vi "11-QNET_MECHKIT_Switches_and_LEDs.vi"() -> ()   [LabVIEW 2017]
doc: "This VI is to be used with the NI-ELVIS and the QNET-Mechatronic Sensors I module. The objective is to calibrate the analog sensors."
uses:
  <vilib>/Simulation/Scripting/Companion Diagram/SimConfigNode/SimParams.ctl
  <vilib>/Simulation/Scripting/Companion Diagram/SimConfigNode/_simSolvers.ctl
  <vilib>/Simulation/Implementation/Shared/SIMSCR Execution Mode.ctl
  <vilib>/Simulation/Param Hierarchy/Typedefs/SIMPH Param Control Actions.ctl
  <vilib>/Simulation/Implementation/Shared/NILVSim_ParamChanged.vi
  <vilib>/Simulation/Implementation/Shared/NILVSIM_BeginStep.vi
  <vilib>/Simulation/SignalDisplay/Implementation/NILVSim Time Waveform.llb/SIM Time Waveform (scalar).vi
  <vilib>/Simulation/Utility/Implementation/SIM Halt.vi
  <vilib>/Simulation/Implementation/Shared/NILVSim_Manager.vi
  <vilib>/Utility/error.llb/Clear Errors.vi
  <vilib>/Simulation/Implementation/Shared/NILVSim_FinalizeModel.vi
  <vilib>/Simulation/Implementation/Shared/SIM Unbundle Sim Info.vi
  <vilib>/Simulation/Implementation/Shared/NILVSim_Initialize.vi
  QNET Library/QNET_Drivers.llb/QNET_MECHKIT_AI_Read.vi
  QNET Library/Quanser_DAQ_MX_Drivers.llb/DO_Write_Multi_MX.vi
  <vilib>/Simulation/Utility/Implementation/NILVSim Get Time and IsAcceptedStep.vi
  <vilib>/Simulation/Implementation/Shared/SIMSH Read Queue.vi
  <vilib>/Simulation/Implementation/Shared/NILVSim_GetModelError.vi
  <vilib>/Simulation/Implementation/Shared/SIM Bundle Sim Info.vi
  <vilib>/Simulation/Scripting/Companion Diagram/SimConfigNode/SimDog.xnode
  <vilib>/Simulation/Implementation/XNodeFramework/SimXNode/SimX.xnode
  <vilib>/Simulation/Implementation/Shared/NI_SIM_Implementation.lvlib
panel:
  in  "Sampling Rate (Hz)":dbl=100.0 min=0.0 max=1000.0 step=25.0 format="%.1f"
  in  "Device":tag="Dev1"
  in  "Tab Control":T1(tab)
  out "Optical Switch":waveform(dbl)(graph)
  out "Optical Switch - Digital":waveform(dbl)(graph)
  in  "Threshold":dbl(slide) min=0.0 max=5.0 step=0.05 scale=0.0..5.0
  out "Micro Switch":waveform(dbl)(graph)
  out "Micro Switch - Digital":waveform(dbl)(graph)
  in  "Gain":dbl step=0.05
  in  "Offset":dbl
  out "Push Button":waveform(dbl)(graph)
  in  "PB Offset":dbl caption="Offset"
  in  "PB Gain":dbl caption="Gain" step=0.05
  out "Push Button - Digital":waveform(dbl)(graph)
  in  "Digital Outputs":cluster{"DO 0":bool, "DO 1":bool}={"DO 0"=TRUE, "DO 1"=FALSE}
  in  "Stop":bool
  # "QNET-Switches and LEDs"
  # "NOTE: Place J7 to \"Opto Switch\", J8 to \"Micro Switch\", and J9 to \"Push Button\"."
  # "s"
  # "1) Take piece of paper and slide it up and down into the optical switch.\n2) Examine the raw responses in the \"Optical Switch\" chart.\n3) Adjust threshold to obtain on/off measurement in the \n\"Optical Switch - Digital\" chart."
  # "if (x > threshold) then y = 1\nelse y = 0"
  # "y = Gain*x + Offset\nwhere:\nx is the switch signal\ny is the processed switch signal"
  # "1) Press on Mirco Switch and examine response in \"Micro Switch\" scope.\n2) Adjust the Gain and Offset such that this signal goes from 0 to 1 \nin the \"Micro Switch - Digital\" scope when the Micro Switch is pressed."
  # "y = Gain*x + Offset\nwhere:\nx is the push button signal\ny is the processed signal"
  # "1) Press on Push Button and examine response in \"Push Button\" scope.\n2) Adjust the Gain and Offset such that the signal goes from 0 to 1 in the \n\"Push Button - Digital\" scope when the Push Button is pressed."
  # "Turn switches UP and DOWN and examine response of LEDs QNET-MECHKIT board."
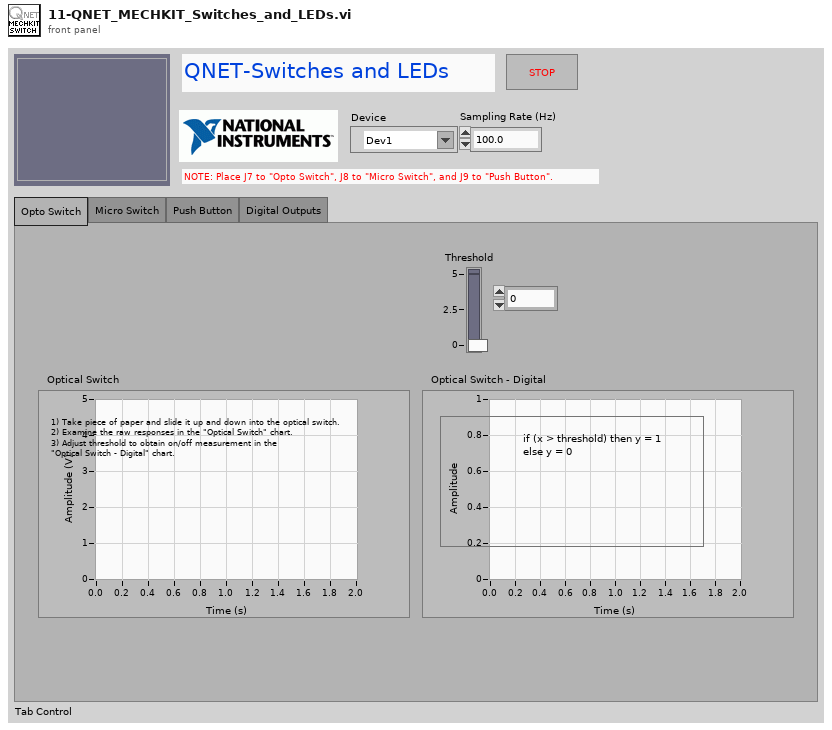
[diagram p1: front panel]
types:
  T1 = enum32{"Opto Switch", "Micro Switch", "Push Button", "Digital Outputs"}
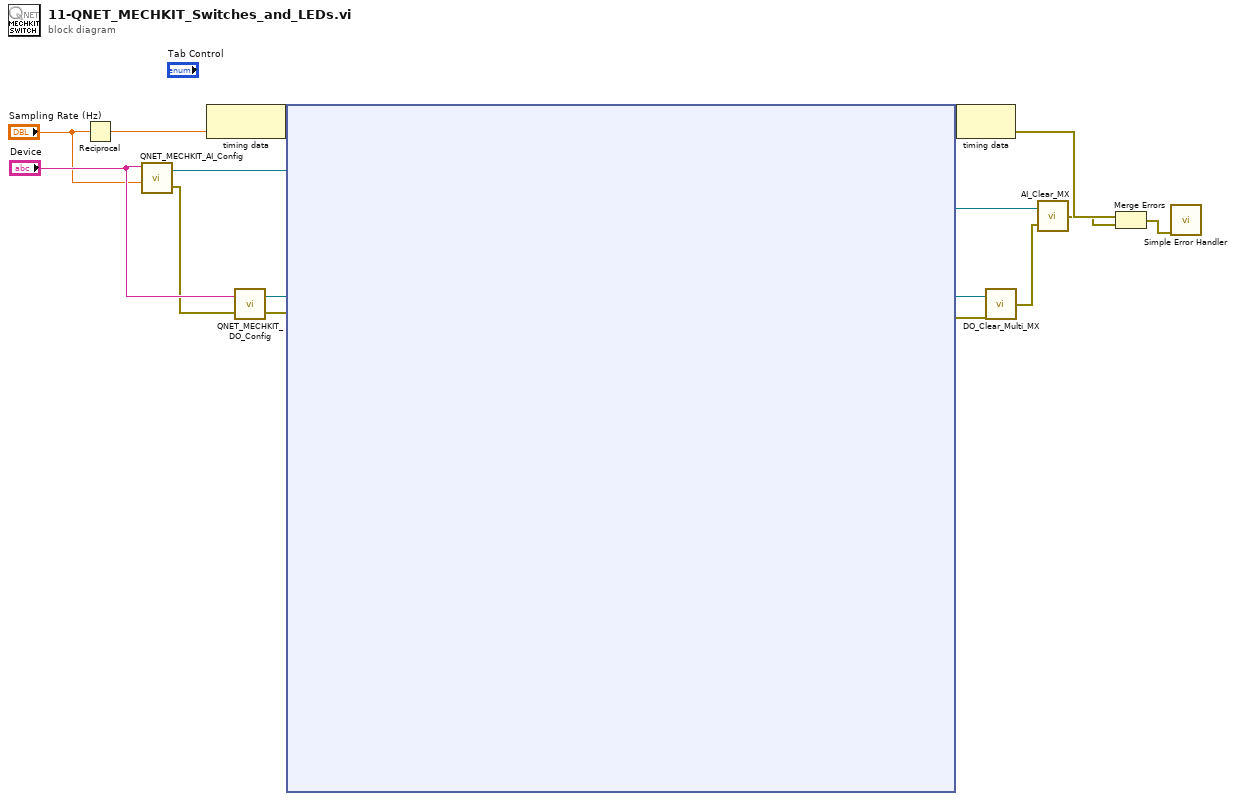
[diagram p0: block diagram]
diagram:
  n1 = Reciprocal(x="Sampling Rate (Hz)") -> (1/x=w5:dbl)
  n2 = call "QNET_MECHKIT_AI_Config.vi"("sampling rate (Hz)"="Sampling Rate (Hz)", "dev"="Device") -> ("error out"=w9:errorcluster, "task out"=w16:refnum<k21>)  [unwired: 2 in]
  n3 = node-c288(w5) -> (w7:variant)
  n4 = call "QNET_MECHKIT_DO_Config.vi"("error in"=w9, "Device"="Device") -> ("error out"=w14:errorcluster, "task out"=w13:refnum<k21>)
  n5 = node-c254 ("Simulation Loop")(w7, w16, w14, w13) -> (w6:variant, w15:errorcluster, w12:refnum<k21>, w11:refnum<k21>)
  n6 = node-c288(w6) -> (w3:errorcluster)
  n7 = call "DO_Clear_Multi_MX.vi"("Error in"=w15, "Task in"=w12) -> ("Error out"=w8:errorcluster)
  n8 = call "AI_Clear_MX.vi"("Error in"=w8, "Task in"=w11) -> ("Error out"=w2:errorcluster)
  n9 = Merge Errors(w3, w2) -> (w1:errorcluster)
  n10 = call <vilib>:"Simple Error Handler.vi"("error in (no error)"=w1) -> ()  [unwired: 1 in, 8 out]
